vi "Init.vi"(8 "error in (no error)":errorcluster caption="entrée d'erreur (pas d'erreur)", 11 "Class DIO (Default) en entrée":refnum<class "Class Ana NI.lvclass">) -> (0 "error out":errorcluster caption="sortie d'erreur", 3 "Class DIO (Default) en sortie":refnum<class "Class Ana NI.lvclass">)   [LabVIEW 2020, in "Library Instrument & Equipement.lvlib" / "Library Ana.lvlib" / "Class Ana NI.lvclass"]
uses:
  Class Ana NI.lvclass
  C:/Users/ngarcin/OneDrive - Altyor/Standard TB/Class/Ana/Class Ana (Default)/Class Ana (Default).lvclass
  <vilib>/DAQmx/create/channels.llb/DAQmx Create Channel (AI-Voltage-Basic).vi
  <vilib>/DAQmx/configure/timing.llb/DAQmx Timing (Sample Clock).vi
  Class Ana NI.lvclass/Class Ana NI.ctl
  C:/Program Files (x86)/National Instruments/LabVIEW 2020/resource/objmgr/daqmx.rc
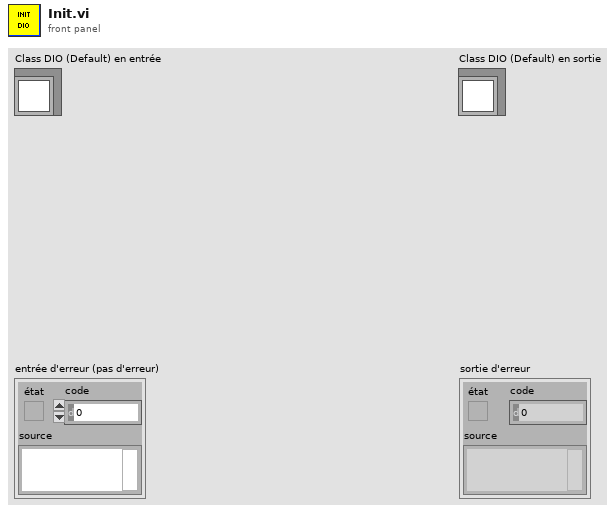
[diagram p1: front panel]
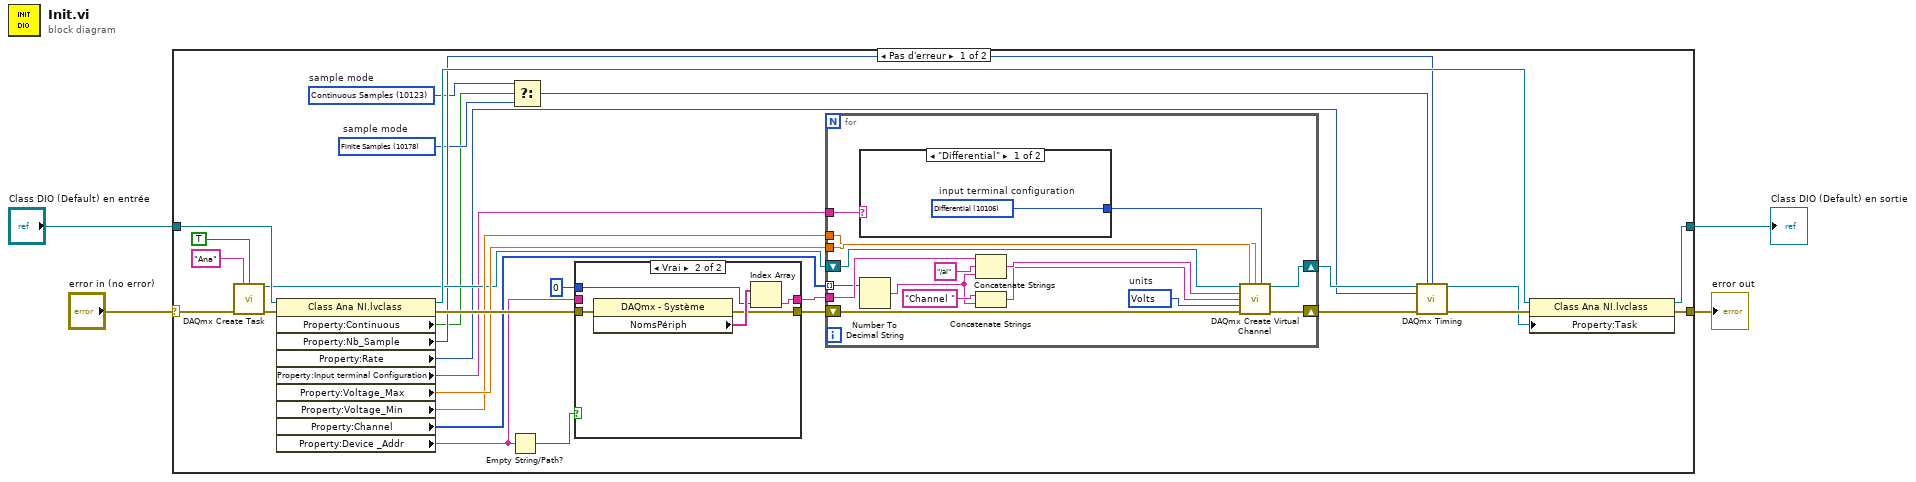
[diagram p0: block diagram]
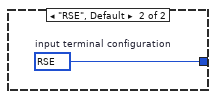
[diagram p2: hidden frame]
diagram:
  n1 = case shown="Pas d'erreur" "error in (no error)" {
    selector: "error in (no error)" -> [w32 w60]
    tunnel: [w25 w60] -> w3
    tunnel: [w24 w59] -> w1
    tunnel: "Class DIO (Default) en entrée" -> [w33 w59]
    frame No Error {
      w6 = 10123 items=["Finite Samples"=10178, "Continuous Samples"=10123, "Hardware Timed Single Point"=12522]  # sample mode
      w8 = 10178 items=["Finite Samples"=10178, "Continuous Samples"=10123, "Hardware Timed Single Point"=12522]  # sample mode
      n2 = call <vilib>:"DAQmx Create Task.vi"("new task name"="Ana", "auto cleanup"=TRUE, "error in"=w32) -> ("task out"=w16:refnum<k21>, "error out"=w31:errorcluster)  [unwired: 11 in]
      n3 = property class="Class Ana NI.lvclass"(reference=w33, error in=w31) -> (reference out=w26:refnum<class "Class Ana NI.lvclass">, error out=w29:errorcluster, "Property:Continuous"=w7:bool, "Property:Nb_Sample"=w12:u16, "Property:Rate"=w11:u16, "Property:Input terminal Configuration"=w10:string, "Property:Voltage_Max"=w18:dbl, "Property:Voltage_Min"=w17:dbl, "Property:Channel"=w19:u8[], "Property:Device _Addr"=w27:string)
      n4 = Empty String/Path?(string/path=w27) -> (empty?=w28:bool)
      n5 = Select(t=w6, s=w7, f=w8) -> (s? t:f=w5:i32)
      n6 = case shown="Vrai" w28 {
        tunnel: 0 ("indice") -> [_ w57]
        tunnel: w29 -> [w53 w56]
        tunnel: [w53 w55] -> w15
        tunnel: [w52 w54] -> w20
        tunnel: w27 -> [w52 _]
        frame False {
        }
        frame True {
          n7 = property class="DAQmx - Système"(error in=w56) -> (error out=w55:errorcluster, "NomsPériph"=w58:tag[])  [unwired: 1 in, 1 out]
          n8 = Index Array(array=w58, index=w57) -> (element=w54:tag)
        }
      }
      n9 = for {
        tunnel: w20 -> [w49]
        tunnel: w19 -> [w47] mode=indexing
        tunnel: w18 -> [w35]
        tunnel: w17 -> [w34]
        shift-right: [w39] -> w13
        shift-left: w15 -> [w40]
        shift-right: [w38] -> w14
        shift-left: w16 -> [w41]
        tunnel: w10 -> [w37]
        w42 = 10348 items=["Volts"=10348, "From Custom Scale"=10065]  # units
        n10 = case shown="\"Differential\"" w37 {
          tunnel: [w50 w51] -> w36
          frame "Differential" {
            w50 = 10106 items=["default"=-1, "RSE"=10083, "NRSE"=10078, "Differential"=10106, "Pseudodifferential"=12529]  # input terminal configuration
          }
          frame "RSE", Default {
            w51 = 10083 items=["default"=-1, "RSE"=10083, "NRSE"=10078, "Differential"=10106, "Pseudodifferential"=12529]  # input terminal configuration
          }
        }
        n11 = Number To Decimal String(number=w47) -> (decimal integer string=w44:string)  [unwired: 1 in]
        n12 = Concatenate Strings(w49, "/ai" ("chaîne"), w44) -> (w46:string)
        n13 = Concatenate Strings("Channel " ("chaîne"), w44) -> (w43:string)
        n14 = call-poly <vilib>:"DAQmx Create Virtual Channel.vi"("task in"=w41, "maximum value"=w35, "minimum value"=w34, "input terminal configuration"=w36, "physical channels"=w46, "name to assign"=w43, "units"=w42, "error in"=w40) -> ("task out"=w38:refnum<k21>, "error out"=w39:errorcluster)  [unwired: 6 in]
      }
      n15 = call-poly <vilib>:"DAQmx Timing.vi"("task/channels in"=w14, "sample mode"=w5, "samples per channel"=w12, "rate"=w11, "error in"=w13) -> ("task out"=w9:refnum<k21>, "error out"=w21:errorcluster)  [unwired: 9 in]
      n16 = property class="Class Ana NI.lvclass"(reference=w26, error in=w21, "Property:Task"=w9) -> (reference out=w24:refnum<class "Class Ana NI.lvclass">, error out=w25:errorcluster)
    }
    frame Error {
    }
  }
  "error out" <- w3
  "Class DIO (Default) en sortie" <- w1
